vi "BaudDetect-Format Line.vi"(10 "Information":cluster{"T0":u8, "T1":u8, "br_selfdef":T1} {"br_selfdef"."PHSEG2" items=["CAN_BIT_1TQ"=1, "CAN_BIT_2TQ"=2, "CAN_BIT_3TQ"=3, "CAN_BIT_4TQ"=4, "CAN_BIT_5TQ"=5, "CAN_BIT_6TQ"=6, "CAN_BIT_7TQ"=7, "CAN_BIT_8TQ"=8]; "br_selfdef"."PHSEG1" items=["CAN_BIT_1TQ"=1, "CAN_BIT_2TQ"=2, "CAN_BIT_3TQ"=3, "CAN_BIT_4TQ"=4, "CAN_BIT_5TQ"=5, "CAN_BIT_6TQ"=6, "CAN_BIT_7TQ"=7, "CAN_BIT_8TQ"=8]; "br_selfdef"."PRSEG" items=["CAN_BIT_1TQ"=1, "CAN_BIT_2TQ"=2, "CAN_BIT_3TQ"=3, "CAN_BIT_4TQ"=4, "CAN_BIT_5TQ"=5, "CAN_BIT_6TQ"=6, "CAN_BIT_7TQ"=7, "CAN_BIT_8TQ"=8]; "br_selfdef"."PHS2_SEL" items=["由相位缓冲段1时间指定", "可编程"]; "br_selfdef"."SAM" items=["采样一次", "采样三次"]; "br_selfdef"."BRP" items=["1"=1, "2"=2, "3"=3, "4"=4, "5"=5, "6"=6, "7"=7, "8"=8, "9"=9, "10"=10, "11"=11, "12"=12, "13"=13, "14"=14, "15"=15, "16"=16, "17"=17, "18"=18, "19"=19, "20"=20, "21"=21, "22"=22, "23"=23, "24"=24, "25"=25, "26"=26, "27"=27, "28"=28, "29"=29, "30"=30, "31"=31, "32"=32, "33"=33, "34"=34, "35"=35, "36"=36, "37"=37, "38"=38, "39"=39, "40"=40, "41"=41, "42"=42, "43"=43, "44"=44, "45"=45, "46"=46, "47"=47, "48"=48, "49"=49, "50"=50, "51"=51, "52"=52, "53"=53, "54"=54, "55"=55, "56"=56, "57"=57, "58"=58, "59"=59, "60"=60, "61"=61, "62"=62, "63"=63, "64"=64]; "br_selfdef"."SJW" items=["1TQ"=1, "2TQ"=2, "3TQ"=3, "4TQ"=4]; "br_selfdef"."SYN(nouse)" items=["CAN_BIT_1TQ"=1]}, 11 "Status":string) -> (3 "Line Array":string[](array[string]))   [LabVIEW 2011]
uses:
  Baud rate Self Define.ctl
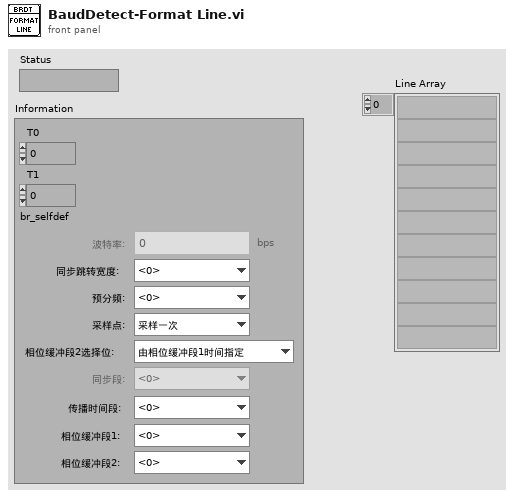
[diagram p1: front panel]
types:
  T1 = typedef "Baud rate Self Define.ctl" = cluster{"BAUD":u32, "SJW":u8, "BRP":u8, "SAM":u8, "PHS2_SEL":u8, "SYN(nouse)":u8, "PRSEG":u8, "PHSEG1":u8, "PHSEG2":u8}
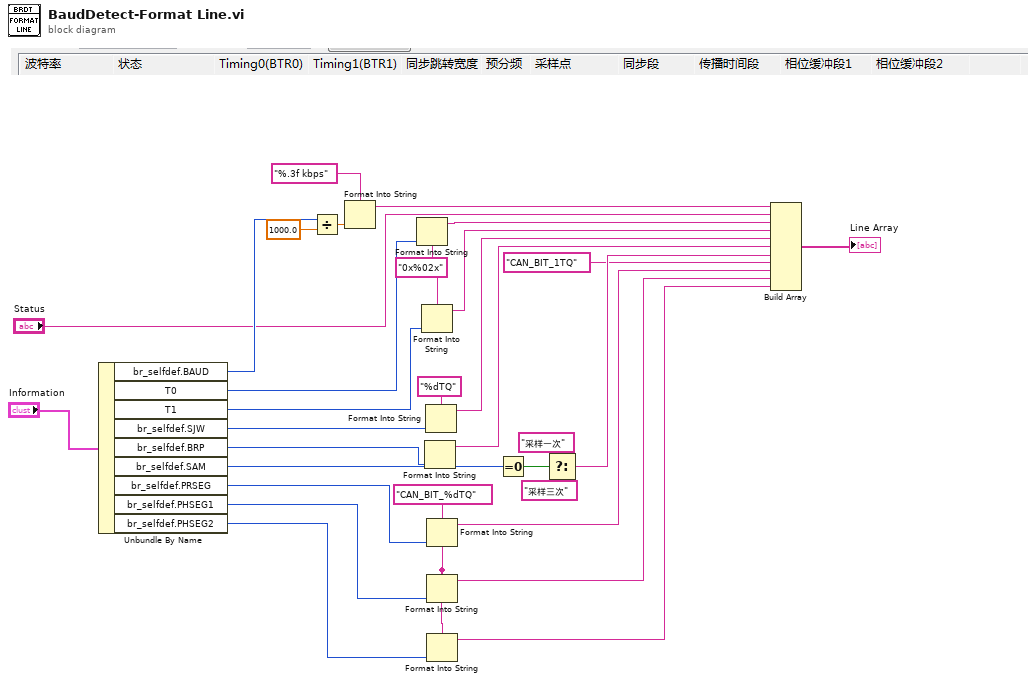
[diagram p0: block diagram]
diagram:
  w4 = "CAN_BIT_%dTQ" ("格式字符串")
  w22 = "0x%02x" ("格式字符串")
  n1 = Unbundle By Name("Information") -> ("br_selfdef.BAUD"=w30:u32, "T0"=w24:u8, "T1"=w21:u8, "br_selfdef.SJW"=w19:u8, "br_selfdef.BRP"=w16:u8, "br_selfdef.SAM"=w14:u8, "br_selfdef.PRSEG"=w8:u8, "br_selfdef.PHSEG1"=w6:u8, "br_selfdef.PHSEG2"=w3:u8)
  n2 = Divide(x=w30, y=1000.0) -> (x/y=w28:dbl)
  n3 = Format Into String(format string="%.3f kbps" ("格式字符串"), w28) -> (resulting string=w26:string)  [unwired: 2 in, 1 out]
  n4 = Format Into String(format string=w22, w24) -> (resulting string=w23:string)  [unwired: 2 in, 1 out]
  n5 = Format Into String(format string=w22, w21) -> (resulting string=w20:string)  [unwired: 2 in, 1 out]
  n6 = Format Into String(w16) -> (resulting string=w15:string)  [unwired: 3 in, 1 out]
  n7 = Format Into String(format string="%dTQ" ("格式字符串"), w19) -> (resulting string=w17:string)  [unwired: 2 in, 1 out]
  n8 = Format Into String(format string=w4, w8) -> (resulting string=w7:string)  [unwired: 2 in, 1 out]
  n9 = Format Into String(format string=w4, w6) -> (resulting string=w5:string)  [unwired: 2 in, 1 out]
  n10 = Format Into String(format string=w4, w3) -> (resulting string=w2:string)  [unwired: 2 in, 1 out]
  n11 = Equal To 0?(x=w14) -> (x = 0?=w13:bool)
  n12 = Select(t="采样一次", s=w13, f="采样三次") -> (s? t:f=w10:string)
  n13 = Build Array(w26, "Status", w23, w20, w17, w15, w10, "CAN_BIT_1TQ", w7, w5, w2) -> (→"Line Array":string[])
